vi "Example-Controller.vi"() -> ()   [LabVIEW 2011]
uses:
  TypeDefs/ExecutionType.ctl
  UI_Interaction_Manager.lvclass
panel:
  in  "stop":bool
  in  "Execution Type":T1
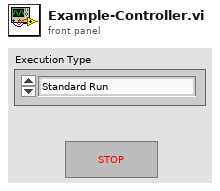
[diagram p1: front panel]
types:
  T1 = typedef "UI_Interaction_Manager.lvclass/ExecutionType.ctl" = enum16{"Standard Run", "Run with Recording", "Auto-Run with Playback"}
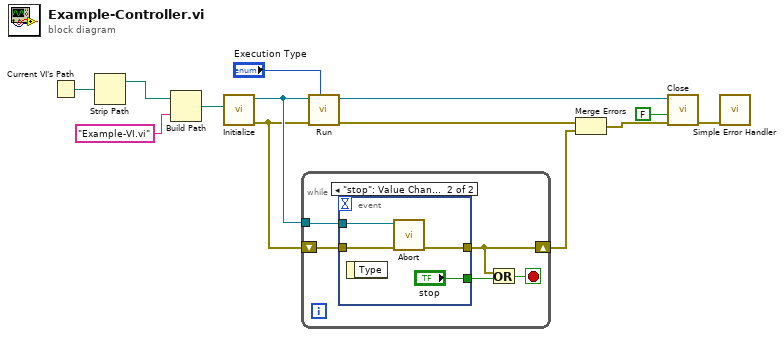
[diagram p0: block diagram]
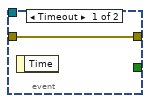
[diagram p2: hidden frame]
diagram:
  n1 = Current VI's Path() -> (path=w2:path)
  n2 = Strip Path(path=w2) -> (stripped path=w1:path)  [unwired: 1 out]
  n3 = Build Path(base path=w1, name or relative path="Example-VI.vi") -> (appended path=w3:path)
  n4 = call "Initialize.vi"("VI Filepath"=w3) -> ("error out"=w6:errorcluster, "UI_Interaction_Manager out"=w11:refnum<class "UI_Interaction_Manager.lvclass">)  [unwired: 9 in]
  n5 = while {
    tunnel: w11 -> [w18]
    shift-right: [w15] -> w7
    shift-left: w6 -> [w17]
    stop <- w14 stop-if-true
    n6 = event shown="[1] \"stop\": Value Change" {
      selector: _ -> [_ _]
      dyn-events: _ -> [_ _]
      timeout: _ -> [_ _]
      tunnel: [_ "stop"] -> w16
      tunnel: w18 -> [_ w22]
      tunnel: [w19 w21] -> w15
      tunnel: w17 -> [w19 w20]
      event Timeout {
        n7 = event-data() -> ()  [unwired: 1 in, 1 out]
      }
      event "stop": Value Change {
        n8 = event-data() -> ()  [unwired: 1 in, 1 out]
        n9 = call "Abort.vi"("error in (no error)"=w20, "UI_Interaction_Manager in"=w22) -> ("error out"=w21:errorcluster)  [unwired: 8 in, 1 out]
      }
    }
    n10 = Or(x=w15, y=w16) -> (x .or. y?=w14:bool)
  }
  n11 = call "Run.vi"("Execution Type"="Execution Type", "error in (no error)"=w6, "UI_Interaction_Manager in"=w11) -> ("error out"=w8:errorcluster, "UI_Interaction_Manager out"=w12:refnum<class "UI_Interaction_Manager.lvclass">)  [unwired: 7 in]
  n12 = Merge Errors(w8, w7) -> (w9:errorcluster)
  n13 = call "Close.vi"("error in (no error)"=w9, "Close after execution (F)?"=FALSE, "UI_Interaction_Manager in"=w12) -> ("error out"=w5:errorcluster)  [unwired: 8 in]
  n14 = call <vilib>:"Simple Error Handler.vi"("error in (no error)"=w5) -> ()  [unwired: 4 in, 5 out]
